vi "Switch Schedule FGV.vi"(7 "Action":T5, 8 "error in (no error)":errorcluster, 9 "Switch Schedule":T4, 10 "Switch Program":T1) -> (0 "error out":errorcluster, 2 "Switch Schedule":T4)   [LabVIEW 2014]
doc: "Functional Global Variable used to maintain the Switch Schedule."
uses:
  Controls/Switch Schedule FGV.ctl
  Controls/Switch Schedule.ctl
  Controls/Switch Program.ctl
  Controls/Action Enum.ctl
  Controls/Switch Day.ctl
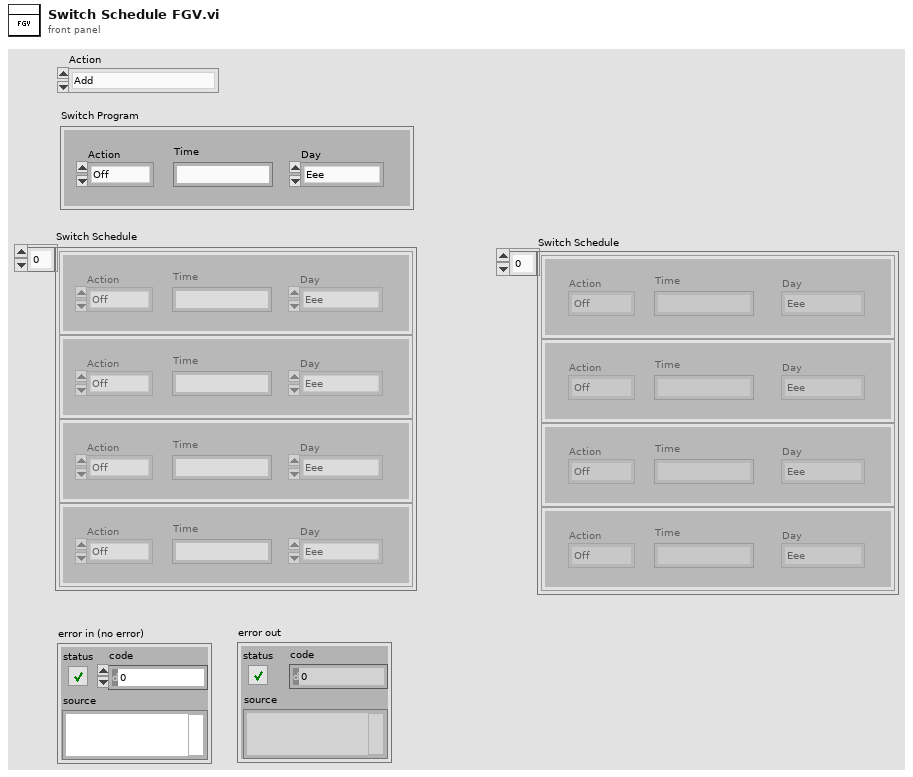
[diagram p1: front panel]
types:
  T1 = typedef "Switch Program.ctl" = cluster{"Action":T2, "Time":string, "Day":T3}
  T2 = typedef "Action Enum.ctl" = enum16{"Off", "On"}
  T3 = typedef "Switch Day.ctl" = enum16{"Eee", "Sun", "Mon", "Tue", "Wed", "Thu", "Fri", "Sat"}
  T4 = typedef "Switch Schedule.ctl" = T1[]
  T5 = typedef "Switch Schedule FGV.ctl" = enum16{"Add", "Delete", "Set", "Get", "Load", "Clear"}
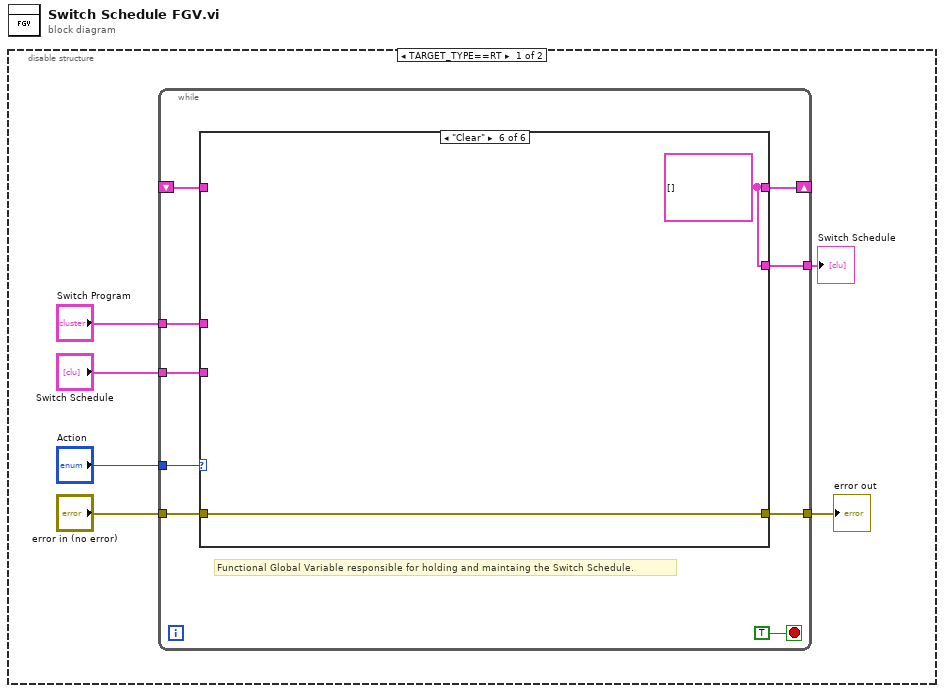
[diagram p0: block diagram]
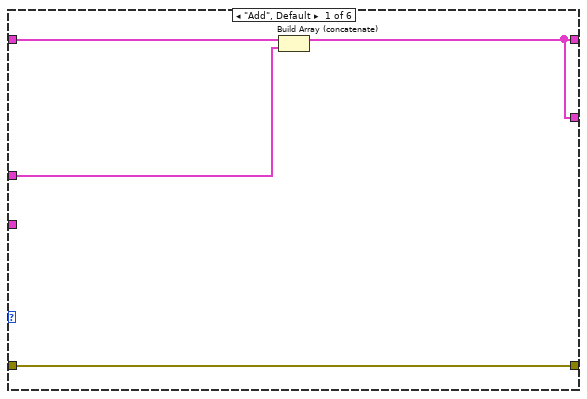
[diagram p2: hidden frame]
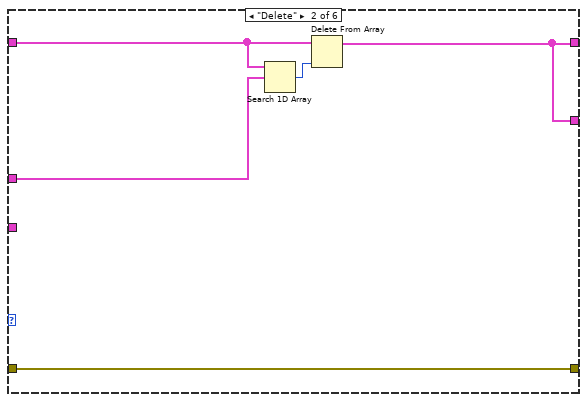
[diagram p3: hidden frame]
diagram:
  n1 = disable-structure shown="TARGET_TYPE==RT" {
    frame condition #0 (active) {
      n2 = while {
        tunnel: "Action" -> [w14]
        shift-right: [w11] -> _
        shift-left: _ -> [w13]
        tunnel: "Switch Schedule" -> [w12]
        tunnel: [w10] -> w4
        tunnel: "Switch Program" -> [w9]
        tunnel: "error in (no error)" -> [w8]
        tunnel: [w7] -> w1
        stop <- TRUE stop-if-true
        # "Functional Global Variable responsible for holding and maintaing the Switch Schedule."
        n3 = case shown="\"Clear\"" w14 {
          tunnel: w13 -> [w19 w23 _ w28 w29 _]
          tunnel: w12 -> [_ _ w26 _ _ _]
          tunnel: [w17 w21 w26 w28 w29 w31] -> w11
          tunnel: [w17 w21 w26 w28 w29 w31] -> w10
          tunnel: w9 -> [w18 w24 _ _ _ _]
          tunnel: w8 -> [w16 w20 w25 w27 w30 w32]
          tunnel: [w16 w20 w25 w27 w30 w32] -> w7
          frame "Add", Default {
            n4 = Build Array (concatenate)(w19, w18) -> (w17:T4)
          }
          frame "Delete" {
            n5 = Search 1D Array(1D array=w23, element=w24) -> (index of element=w22:i32)  [unwired: 1 in]
            n6 = Delete From Array(array=w23, index=w22) -> (array with subset deleted=w21:T4)  [unwired: 1 in, 1 out]
          }
          frame "Set" {
          }
          frame "Get" {
          }
          frame "Load" {
            # "Load Schedule from File"
          }
          frame "Clear" {
            w31 = T4 [] ("Switch Schedule")
          }
        }
      }
      "Switch Schedule" <- w4
      "error out" <- w1
    }
    frame condition #1 {
    }
  }
